vi "Write Map.vi"(8 "error in (no error)":errorcluster, 10 "Map":T1, 11 "Simple Map Queue Group Messenger in":refnum<class "Simple Map Queue Group Messenger.lvclass">) -> (0 "error out":errorcluster, 3 "Simple Map Queue Group Messenger out":refnum<class "Simple Map Queue Group Messenger.lvclass">)   [LabVIEW 2024, in "Simple Map Queue Group Messenger.lvclass"]
uses:
  Simple Map Queue Group Messenger.lvclass
  TypeDef/Queue Group Map.ctl
  Simple Tree Queue Messenger/Type Def/Message Queue.ctl
  Ancestor Class/Message/Message.lvclass
  Simple Map Queue Group Messenger.lvclass/Simple Map Queue Group Messenger.ctl
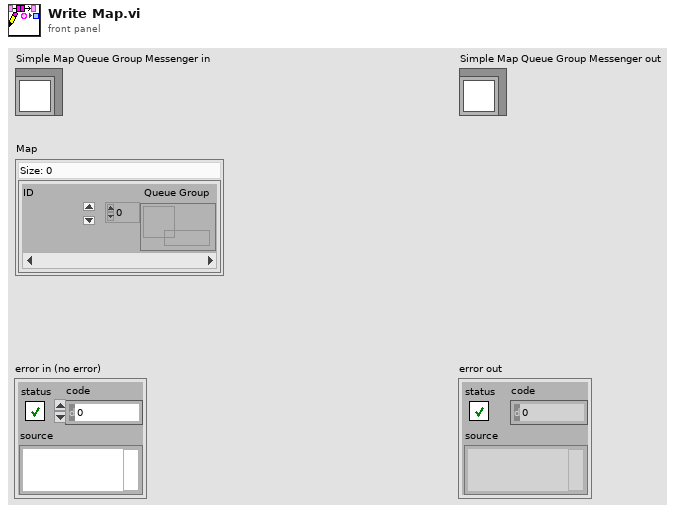
[diagram p1: front panel]
types:
  T1 = typedef "Queue Group Map.ctl" = map{i64, T2[]}
  T2 = typedef "Message Queue.ctl" = refnum<queue>
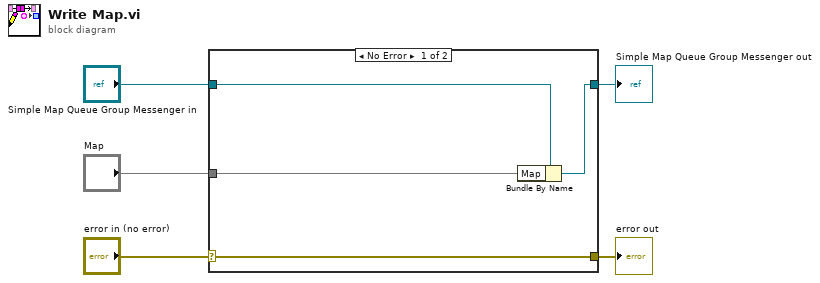
[diagram p0: block diagram]
diagram:
  n1 = case shown="No Error" "error in (no error)" {
    selector: "error in (no error)" -> [w9 w10]
    tunnel: [w9 w10] -> w4
    tunnel: [w7 w11] -> w2
    tunnel: "Simple Map Queue Group Messenger in" -> [w8 w11]
    tunnel: "Map" -> [w6 _]
    frame No Error {
      n2 = Bundle By Name(cluster=w8, "Map"=w6) -> (w7:refnum<class "Simple Map Queue Group Messenger.lvclass">)
    }
    frame Error {
    }
  }
  "error out" <- w4
  "Simple Map Queue Group Messenger out" <- w2
